vi "display_element.vi"(0 "Name":string caption="Enter your name", 5 "place":T3, 7 "cartoon":T2, 9 "color":T1, 11 "error in":errorcluster) -> (8 "path":path, 15 "error out":errorcluster)   [LabVIEW 2023]
uses:
  custom_elements/continue.ctl
  custom_elements/fav_places.ctl
  custom_elements/fav_cartoon.ctl
  custom_elements/fav_colorctl.ctl
panel:
  out "element":string
  in  "stop":T4
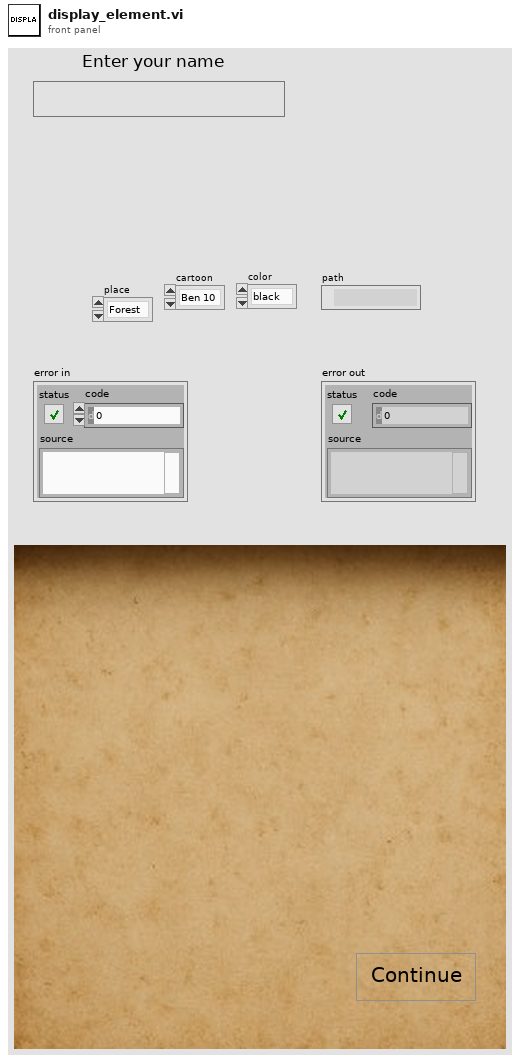
[diagram p1: front panel]
types:
  T1 = typedef "fav_colorctl.ctl" = enum16{"black", "blue", "green", "red"}
  T2 = typedef "fav_cartoon.ctl" = enum16{"Ben 10", "Shin Chan", "Pokemon", "Tom and Jerry"}
  T3 = typedef "fav_places.ctl" = enum16{"Forest", "Mountain", "Beach", "Home"}
  T4 = typedef "continue.ctl" = bool
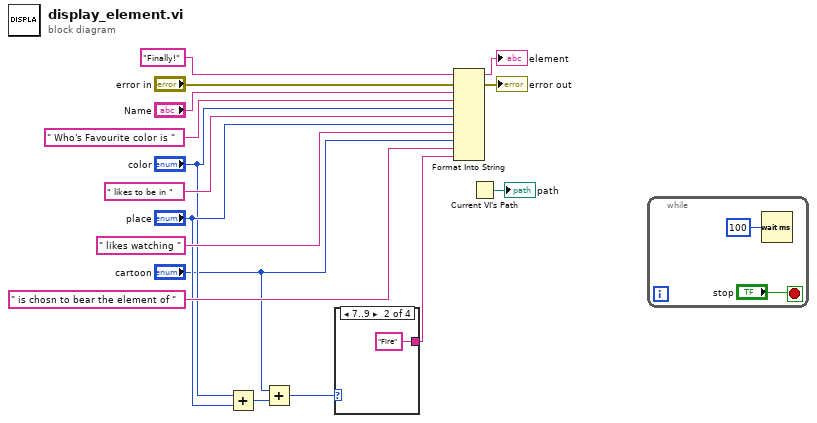
[diagram p0: block diagram]
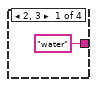
[diagram p2: hidden frame]
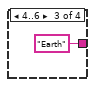
[diagram p3: hidden frame]
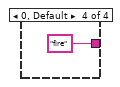
[diagram p4: hidden frame]
diagram:
  n1 = Add(x="color", y="place") -> (x+y=w2:u16)
  n2 = Add(x="cartoon", y=w2) -> (x+y=w1:u16)
  n3 = case shown="7..9" w1 {
    tunnel: ["water" ("input 9") "Fire" ("input 9") "Earth" ("input 9") "fire" ("input 9")] -> w6
    frame 2, 3 {
    }
    frame 7..9 {
    }
    frame 4..6 {
    }
    frame 0, Default {
    }
  }
  n4 = Format Into String(initial string="Finally!", error in="error in", "Name", " Who's Favourite color is " ("input 2"), "color", " likes to be in " ("input 4"), "place", " likes watching " ("input 6"), "cartoon", " is chosn to bear the element of " ("input 8"), w6) -> (resulting string=→"element":string, error out=→"error out":errorcluster)  [unwired: 1 in]
  n5 = Current VI's Path() -> (path=→"path":path)
  n6 = while {
    stop <- "stop" stop-if-true
    n7 = Wait (ms)(milliseconds to wait=u32 100) -> ()  [unwired: 1 out]
  }
